vi "CMWtestsubscribeINT.vi"(8 "error in (no error)":errorcluster, 11 "URL":string="VAC.VGHA_41677/PR") -> (0 "error out":errorcluster, 2 "CMWshort":string, 3 "Numeric":i16)   [LabVIEW 2014]
uses:
  <userlib>/_RADE/RIO/CMW/classes/CMWSubscribe/openCMWSubscribe.vi
  <userlib>/_RADE/RIO/CMW/classes/CMWSubscribe/CMWSubscribe.vi
  <userlib>/_RADE/RIO/CMW/classes/CMWSubscribe/CMWSubscribe.lvclass
panel:
  out "Data":variant
  out "Loop":i32
  in  "stop":bool
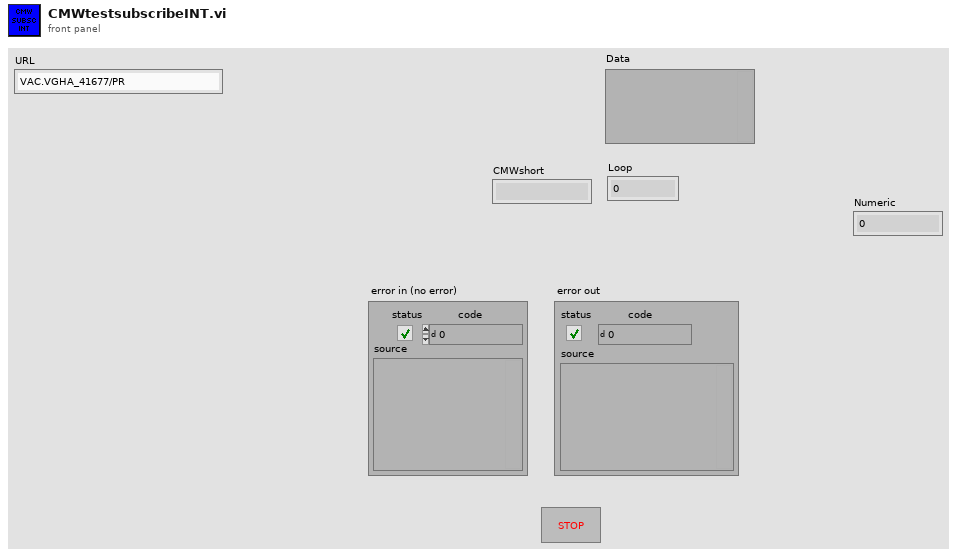
[diagram p1: front panel]
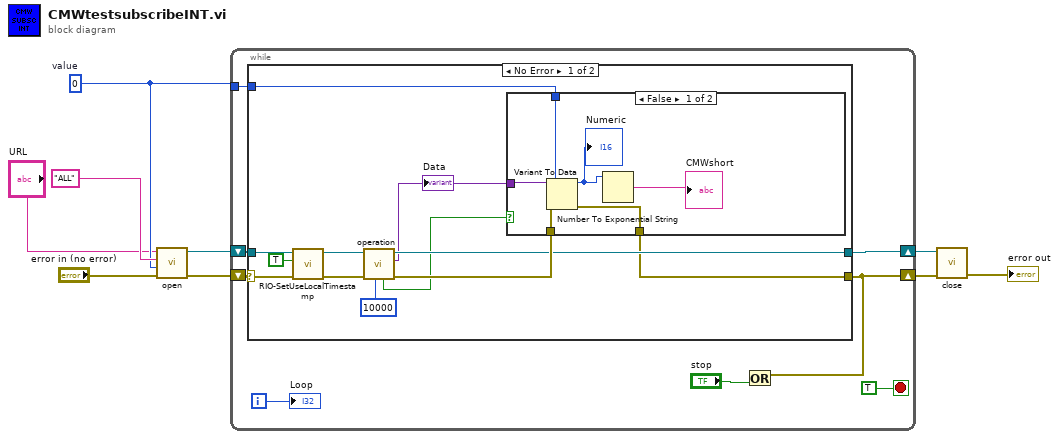
[diagram p0: block diagram]
diagram:
  w2 = i16 0  # value
  n1 = call-poly <userlib>:"open.vi"("error in (no error)"="error in (no error)", "Data type"=w2, "Cycle"="ALL", "URL"="URL") -> ("error out"=w7:errorcluster, "Object out"=w6:refnum<class "CMWSubscribe.lvclass">)  [unwired: 6 in]
  n2 = while {
    shift-right: [w14] -> w5
    shift-left: w7 -> [w17]
    shift-right: [w12] -> w4
    shift-left: w6 -> [w13]
    tunnel: w2 -> [w11]
    i -> [w15]
    stop <- TRUE stop-if-true
    n3 = case shown="No Error" w17 {
      selector: w17 -> [w22 w38]
      tunnel: [w27 w38] -> w14
      tunnel: w13 -> [w20 w37]
      tunnel: [w28 w37] -> w12
      tunnel: w11 -> [w26 _]
      frame No Error {
        n4 = call-dynamic "RIO-SetUseLocalTimestamp.vi"("error in (no error)"=w22, "Use Local Timestamp?"=TRUE, "CMWBase in"=w20) -> ("error out"=w21:errorcluster, "CMWBase out"=w19:refnum<class "CMWSubscribe.lvclass">)  [unwired: 7 in]
        n5 = call-poly <userlib>:"operation.vi"("Timeout (10000 ms)"=10000, "error in (no error)"=w21, "Object in"=w19) -> ("error out"=w29:errorcluster, "Data"=w25:variant, "Object out"=w28:refnum<class "CMWSubscribe.lvclass">, "Timeout?"=w23:bool)  [unwired: 4 in, 1 out]
        "Data" <- w25
        n6 = case shown="False" w23 {
          tunnel: w29 -> [w35 w36]
          tunnel: [w32 w36] -> w27
          tunnel: w25 -> [w34 _]
          tunnel: w26 -> [w33 _]
          frame False {
            n7 = Variant To Data(error in=w35, type=w33, Variant=w34) -> (data=w31:i16, error out=w32:errorcluster)
            "Numeric" <- w31
            n8 = Number To Exponential String(number=w31) -> (E-format string=→"CMWshort":string)  [unwired: 3 in]
          }
          frame True {
          }
        }
      }
      frame Error {
      }
    }
    n9 = Or(x=w14, y="stop") -> ()  [unwired: 1 out]
    "Loop" <- w15
  }
  n10 = call-dynamic "close.vi"("error in (no error)"=w5, "Object in"=w4) -> ("error out"=→"error out":errorcluster)  [unwired: 9 in]
